vi "TurnOff_PowerSupply.vi"(5 "Channel_B":T1, 7 "Channel_A":T1, 8 "error in (no error)":errorcluster {"code" format="%.0x"}, 10 "Keysight PS":bool, 11 "VISA resource name":refnum<visa-resource-name>) -> (0 "error out":errorcluster {"code" format="%.0x"})   [LabVIEW 2018]
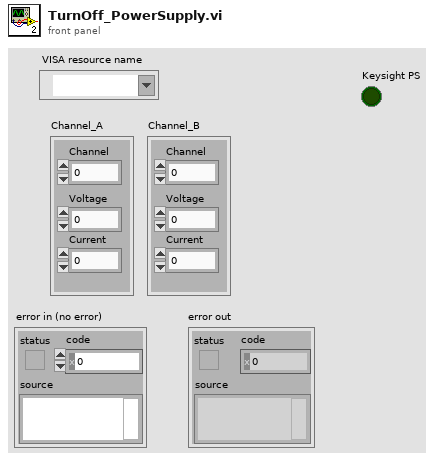
[diagram p1: front panel]
types:
  T1 = cluster{"Channel":dbl, "Voltage":dbl, "Current":dbl}
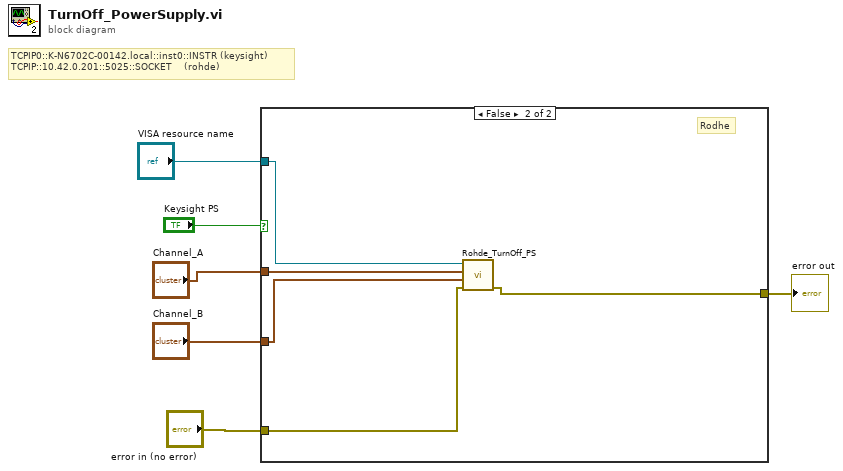
[diagram p0: block diagram]
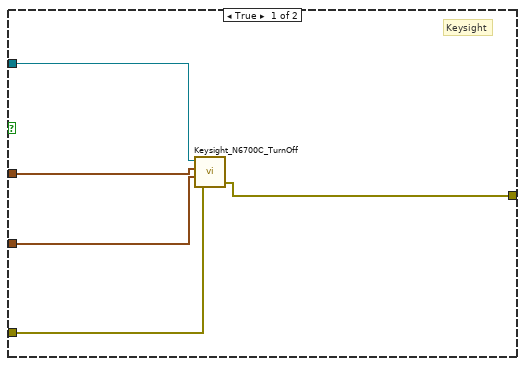
[diagram p2: hidden frame]
diagram:
  # "TCPIP0::K-N6702C-00142.local::inst0::INSTR (keysight)\nTCPIP::10.42.0.201::5025::SOCKET    (rohde)"
  n1 = case shown="False" "Keysight PS" {
    tunnel: "error in (no error)" -> [w9 w16]
    tunnel: [w8 w15] -> w5
    tunnel: "Channel_A" -> [w11 w14]
    tunnel: "Channel_B" -> [w10 w13]
    tunnel: "VISA resource name" -> [w7 w12]
    frame True {
      # "Keysight"
      n2 = call "Keysight_N6700C_TurnOff.vi"("error in (no error)"=w9, "Channel_B"=w10, "Channel_A"=w11, "VISA resource name"=w7) -> ("error out"=w8:errorcluster)  [unwired: 2 in]
    }
    frame False {
      # "Rodhe"
      n3 = call "Rohde_TurnOff_PS.vi"("error in (no error)"=w16, "Channel_B"=w13, "Channel_A"=w14, "VISA resource name"=w12) -> ("error out"=w15:errorcluster)  [unwired: 7 in]
    }
  }
  "error out" <- w5
